vi "Generate Query.vi"(8 "error in (no error)":errorcluster, 11 "Cluster In":T1={"From Date"=timestamp(0 s since 1904-01-01), "To Date"=timestamp(0 s since 1904-01-01), "Selected Database"="", "Selected Table"="", "Selected Field"="", "Field Data"="", "DB Connection Ststus"="", "User Instruction"="", "All/ Top 1000"=FALSE, "Table Data"=[], "Query"="", "Selected Server"="", "Connection Status"=FALSE, "User ID"="", "Password"="", "Date/Field"=FALSE, "(Date/Field/All)"=enum."False", "First Run"=TRUE, "Selected DB Tables"=[], "From Date Field"="", "To Date Field"="", "Selected Table Fields"=[], "Search Type"="", "Reference"={"Top 1000/ All"=refnum, "Search by date"=refnum, "From Date"=refnum, "Select Field"=refnum, "Field Data"=refnum, "To Date"=refnum, "Tables"=refnum, "Search Type"=refnum}, "Mahine RUN Time"=0.0, "Pass/Fail querry"=""}) -> (0 "error out":errorcluster, 3 "Cluster Out":T1={"From Date"=timestamp(0 s since 1904-01-01), "To Date"=timestamp(0 s since 1904-01-01), "Selected Database"="", "Selected Table"="", "Selected Field"="", "Field Data"="", "DB Connection Ststus"="", "User Instruction"="", "All/ Top 1000"=FALSE, "Table Data"=[], "Query"="", "Selected Server"="", "Connection Status"=FALSE, "User ID"="", "Password"="", "Date/Field"=FALSE, "(Date/Field/All)"=enum."False", "First Run"=TRUE, "Selected DB Tables"=[], "From Date Field"="", "To Date Field"="", "Selected Table Fields"=[], "Search Type"="", "Reference"={"Top 1000/ All"=refnum, "Search by date"=refnum, "From Date"=refnum, "Select Field"=refnum, "Field Data"=refnum, "To Date"=refnum, "Tables"=refnum, "Search Type"=refnum}, "Mahine RUN Time"=0.0, "Pass/Fail querry"=""})   [LabVIEW 2017]
uses:
  Controls/Main Cluster.ctl
  Controls/GUI Reference Cluster.ctl
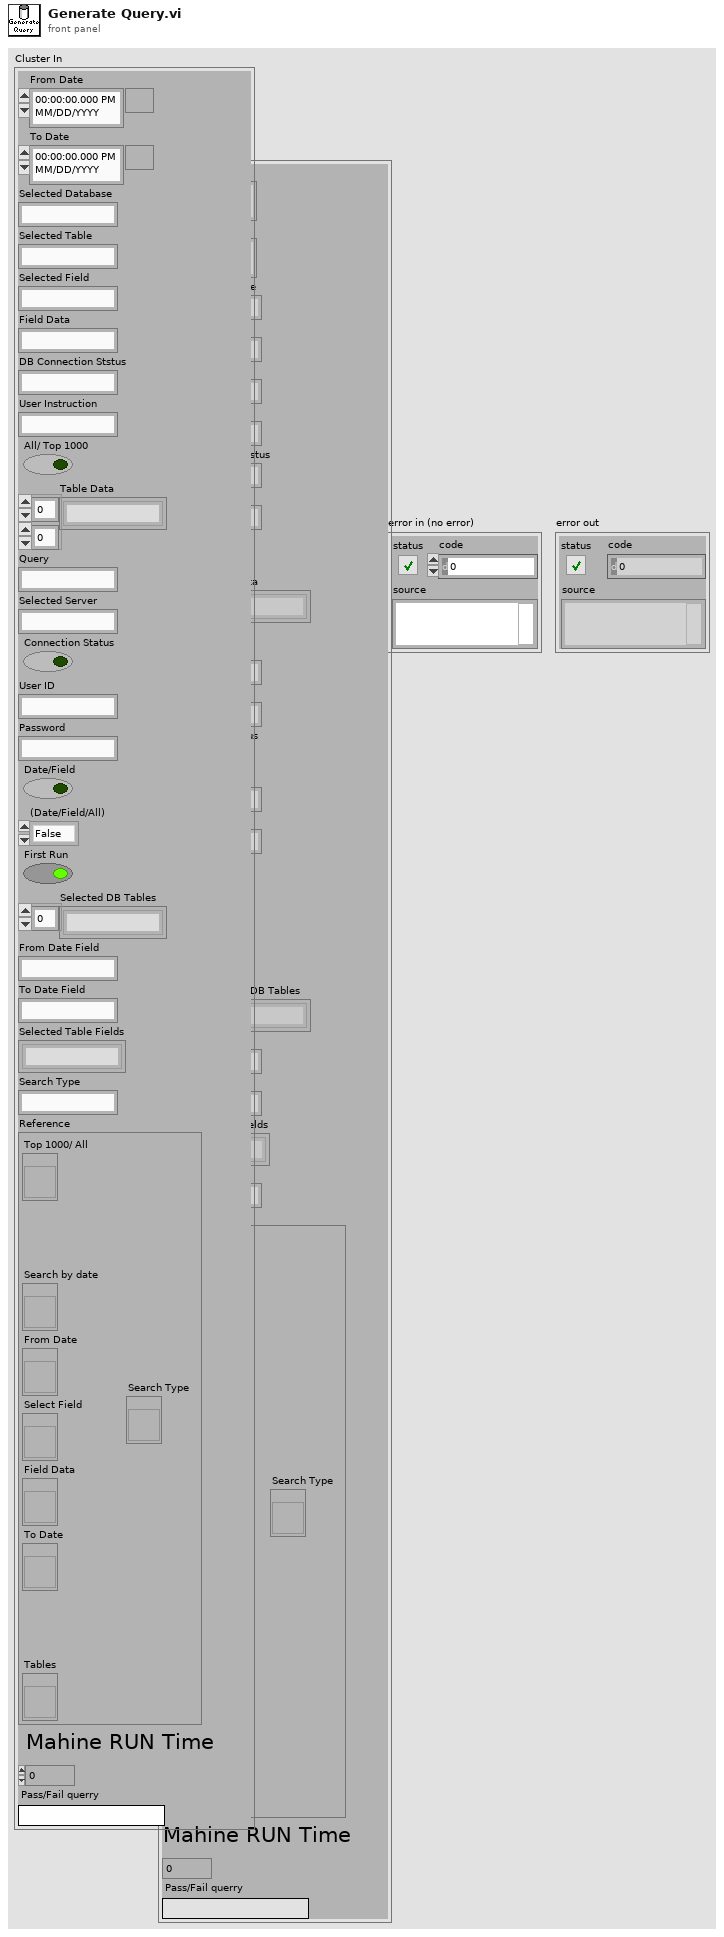
[diagram p1: front panel]
types:
  T1 = typedef "Main Cluster.ctl" = cluster{"From Date":timestamp, "To Date":timestamp, "Selected Database":string, "Selected Table":string, "Selected Field":string, "Field Data":string, "DB Connection Ststus":string, "User Instruction":string, "All/ Top 1000":bool, "Table Data":string[][], "Query":string, "Selected Server":string, "Connection Status":bool, "User ID":string, "Password":string, "Date/Field":bool, "(Date/Field/All)":enum8{"False", "True", "Mixed"}, "First Run":bool, "Selected DB Tables":string[], "From Date Field":string, "To Date Field":string, "Selected Table Fields":string[], "Search Type":string, "Reference":T2, "Mahine RUN Time":dbl, "Pass/Fail querry":string}
  T2 = typedef "GUI Reference Cluster.ctl" = cluster{"Top 1000/ All":refnum<vi>, "Search by date":refnum<vi>, "From Date":refnum<vi>, "Select Field":refnum<vi>, "Field Data":refnum<vi>, "To Date":refnum<vi>, "Tables":refnum<vi>, "Search Type":refnum<vi>}
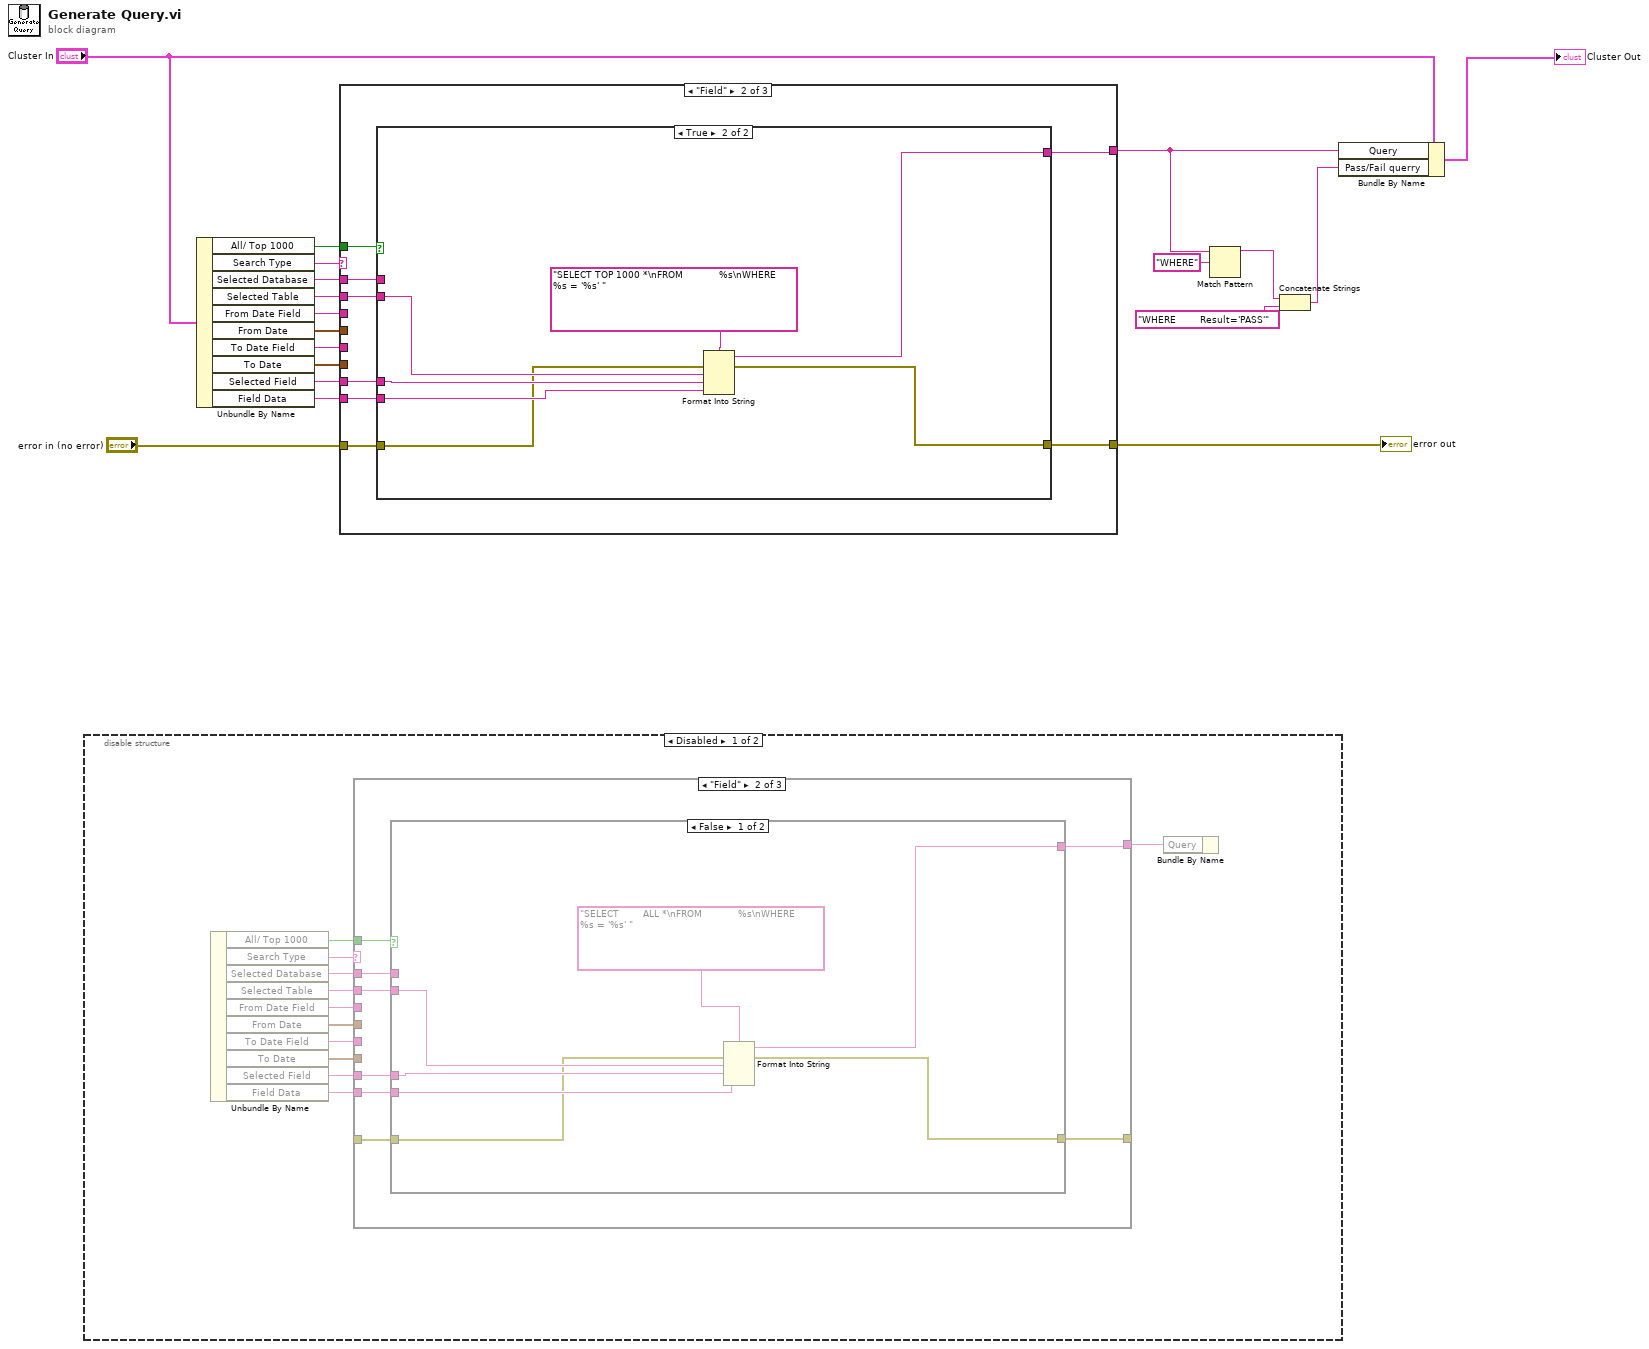
[diagram p0: block diagram]
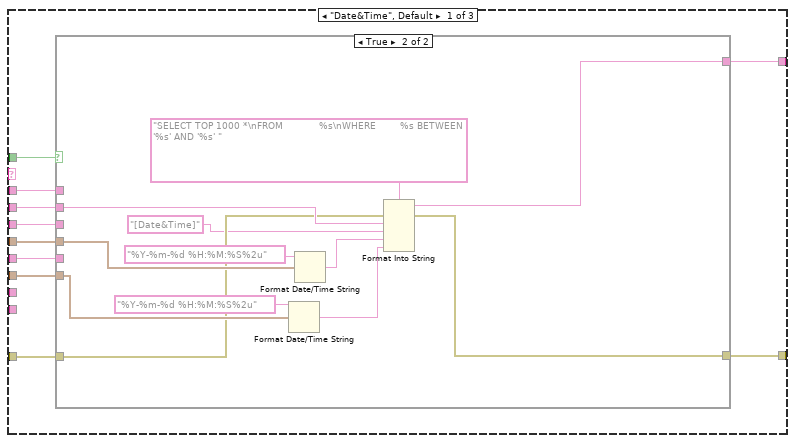
[diagram p2: hidden frame]
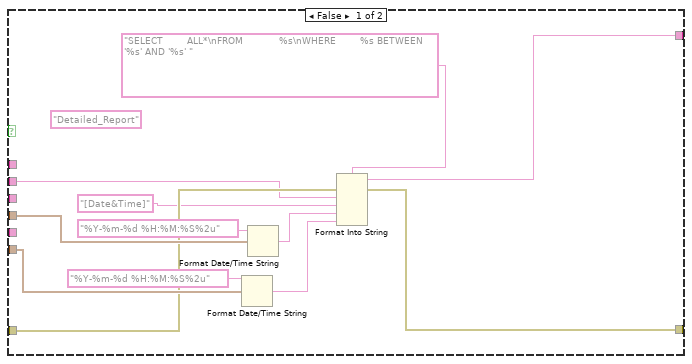
[diagram p3: hidden frame]
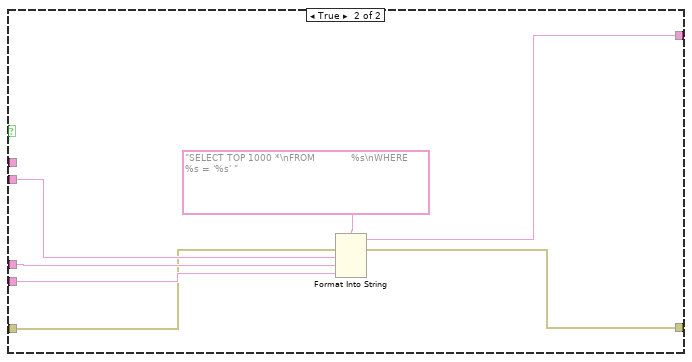
[diagram p4: hidden frame]
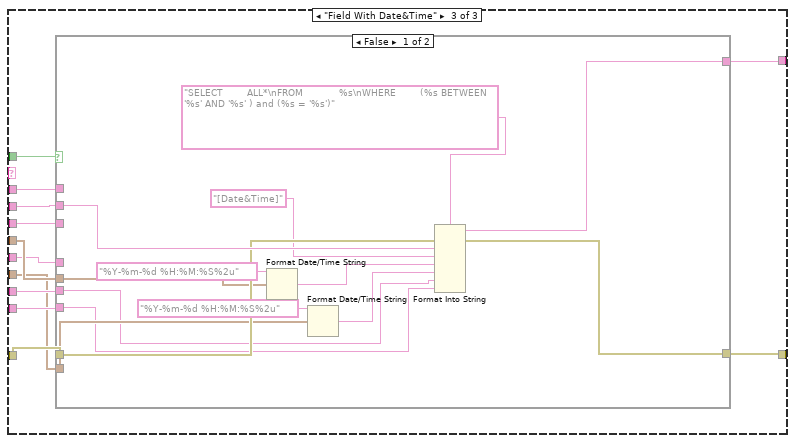
[diagram p5: hidden frame]
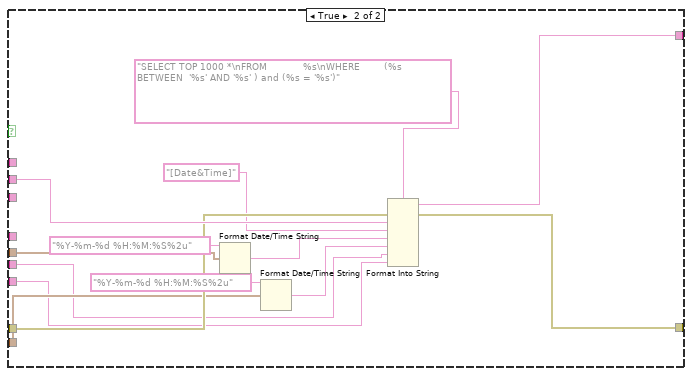
[diagram p6: hidden frame]
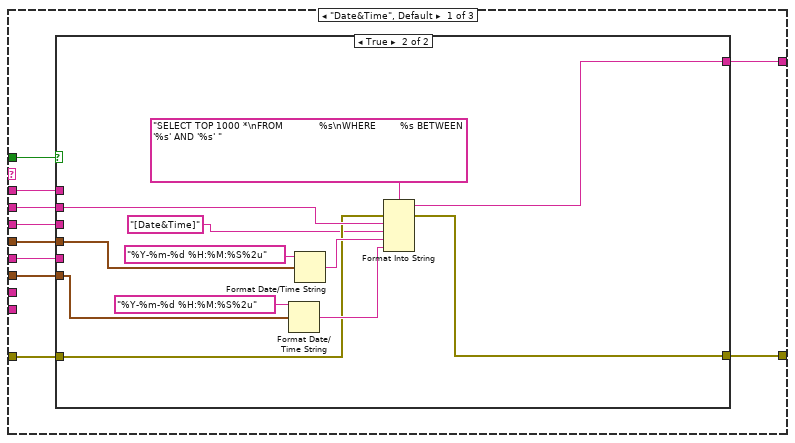
[diagram p8: hidden frame]
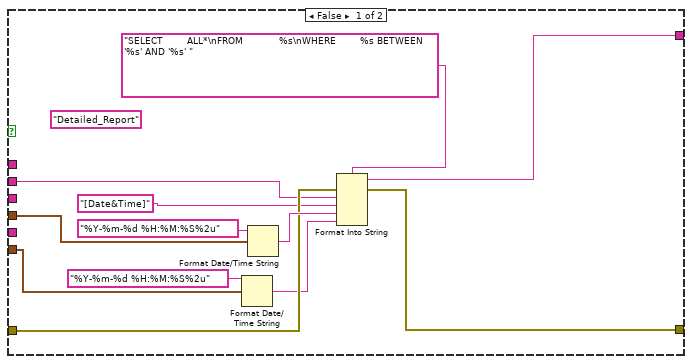
[diagram p9: hidden frame]
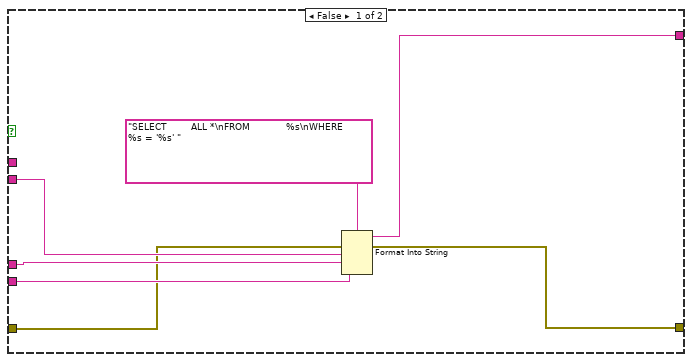
[diagram p10: hidden frame]
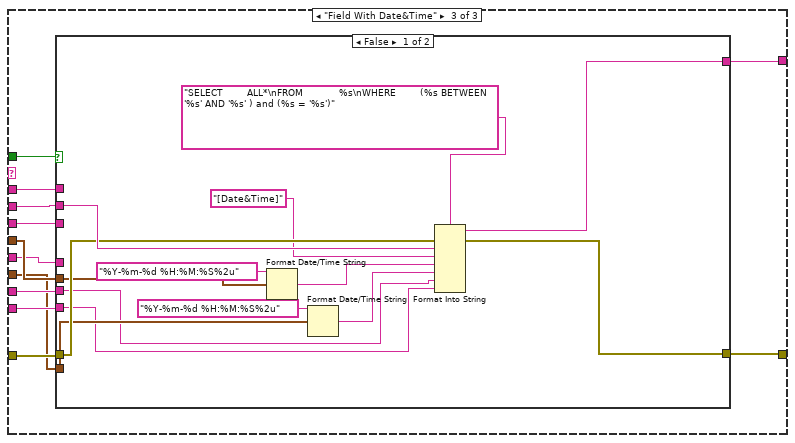
[diagram p11: hidden frame]
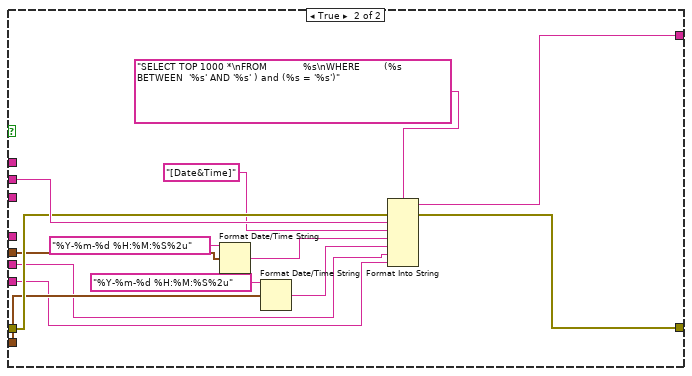
[diagram p12: hidden frame]
diagram:
  n1 = disable-structure shown="Disabled" {
    frame Disabled {
      n2 = Unbundle By Name() -> ("All/ Top 1000"=w21:bool, "Search Type"=w20:string, "Selected Database"=w23:string, "Selected Table"=w24:string, "From Date Field"=w25:string, "From Date"=w26:timestamp, "To Date Field"=w27:string, "To Date"=w28:timestamp, "Selected Field"=w30:string, "Field Data"=w31:string)  [unwired: 1 in]
      n3 = case shown="\"Field\"" w20 {
        tunnel: w21 -> [w42 w70 w98]
        tunnel: w23 -> [w41 w74 w96]
        tunnel: w24 -> [w40 w73 w95]
        tunnel: w25 -> [w39 _ w92]
        tunnel: w26 -> [w38 _ w91]
        tunnel: w27 -> [w37 _ w90]
        tunnel: w28 -> [w36 _ w89]
        tunnel: [w35 w69 w100] -> w29
        tunnel: w30 -> [_ w72 w94]
        tunnel: w31 -> [_ w71 w93]
        tunnel: [w34 w68 w97] -> w32
        tunnel: [w33 w67 w99] -> _
        frame "Date&Time", Default {
          n4 = case shown="True" w42 {
            tunnel: w41 -> [_ _]
            tunnel: w40 -> [w43 w66]
            tunnel: w39 -> [_ _]
            tunnel: w38 -> [w54 w65]
            tunnel: w37 -> [_ _]
            tunnel: w36 -> [w50 w61]
            tunnel: [w49 w59] -> w35
            tunnel: w34 -> [w48 w58]
            tunnel: [w47 w57] -> w33
            frame False {
              (unwired) "Detailed_Report"
              n5 = Format Date/Time String(time format string (%c)="%Y-%m-%d %H:%M:%S%2u", seconds (now)=w50) -> (date/time string=w44:string)  [unwired: 1 in]
              n6 = Format Date/Time String(time format string (%c)="%Y-%m-%d %H:%M:%S%2u", seconds (now)=w54) -> (date/time string=w52:string)  [unwired: 1 in]
              n7 = Format Into String(format string="SELECT        ALL*\nFROM            %s\nWHERE        %s BETWEEN  '%s' AND '%s' ", error in=w48, w43, "[Date&Time]", w52, w44) -> (resulting string=w49:string, error out=w47:errorcluster)  [unwired: 1 in]
            }
            frame True {
              n8 = Format Date/Time String(time format string (%c)="%Y-%m-%d %H:%M:%S%2u", seconds (now)=w61) -> (date/time string=w60:string)  [unwired: 1 in]
              n9 = Format Date/Time String(time format string (%c)="%Y-%m-%d %H:%M:%S%2u", seconds (now)=w65) -> (date/time string=w63:string)  [unwired: 1 in]
              n10 = Format Into String(format string="SELECT TOP 1000 *\nFROM            %s\nWHERE        %s BETWEEN  '%s' AND '%s' ", error in=w58, w66, "[Date&Time]", w63, w60) -> (resulting string=w59:string, error out=w57:errorcluster)  [unwired: 1 in]
            }
          }
        }
        frame "Field" {
          n11 = case shown="False" w70 {
            tunnel: [w81 w88] -> w69
            tunnel: w74 -> [_ _]
            tunnel: w73 -> [w80 w87]
            tunnel: w72 -> [w79 w86]
            tunnel: w71 -> [w78 w85]
            tunnel: w68 -> [w77 w84]
            tunnel: [w76 w83] -> w67
            frame False {
              n12 = Format Into String(format string="SELECT        ALL *\nFROM            %s\nWHERE        %s = '%s' ", error in=w77, w80, w79, w78) -> (resulting string=w81:string, error out=w76:errorcluster)  [unwired: 1 in]
            }
            frame True {
              n13 = Format Into String(format string="SELECT TOP 1000 *\nFROM            %s\nWHERE        %s = '%s' ", error in=w84, w87, w86, w85) -> (resulting string=w88:string, error out=w83:errorcluster)  [unwired: 1 in]
            }
          }
        }
        frame "Field With Date&Time" {
          n14 = case shown="False" w98 {
            tunnel: [w114 w128] -> w100
            tunnel: w96 -> [_ _]
            tunnel: w95 -> [w113 w127]
            tunnel: w94 -> [w102 w116]
            tunnel: w93 -> [w101 w115]
            tunnel: w97 -> [w112 w126]
            tunnel: [w111 w125] -> w99
            tunnel: w92 -> [_ _]
            tunnel: w91 -> [w110 w124]
            tunnel: w90 -> [_ _]
            tunnel: w89 -> [w106 w120]
            frame False {
              n15 = Format Date/Time String(time format string (%c)="%Y-%m-%d %H:%M:%S%2u", seconds (now)=w110) -> (date/time string=w108:string)  [unwired: 1 in]
              n16 = Format Date/Time String(time format string (%c)="%Y-%m-%d %H:%M:%S%2u", seconds (now)=w106) -> (date/time string=w105:string)  [unwired: 1 in]
              n17 = Format Into String(format string="SELECT        ALL*\nFROM            %s\nWHERE        (%s BETWEEN  '%s' AND '%s' ) and (%s = '%s')", error in=w112, w113, "[Date&Time]", w108, w105, w102, w101) -> (resulting string=w114:string, error out=w111:errorcluster)  [unwired: 1 in]
            }
            frame True {
              n18 = Format Date/Time String(time format string (%c)="%Y-%m-%d %H:%M:%S%2u", seconds (now)=w124) -> (date/time string=w122:string)  [unwired: 1 in]
              n19 = Format Date/Time String(time format string (%c)="%Y-%m-%d %H:%M:%S%2u", seconds (now)=w120) -> (date/time string=w119:string)  [unwired: 1 in]
              n20 = Format Into String(format string="SELECT TOP 1000 *\nFROM            %s\nWHERE        (%s BETWEEN  '%s' AND '%s' ) and (%s = '%s')", error in=w126, w127, "[Date&Time]", w122, w119, w116, w115) -> (resulting string=w128:string, error out=w125:errorcluster)  [unwired: 1 in]
            }
          }
        }
      }
      n21 = Bundle By Name("Query"=w29) -> (w22:cluster{})  [unwired: 1 out]
    }
    frame Enabled {
    }
  }
  n22 = Unbundle By Name("Cluster In") -> ("All/ Top 1000"=w18:bool, "Search Type"=w19:string, "Selected Database"=w16:string, "Selected Table"=w15:string, "From Date Field"=w14:string, "From Date"=w13:timestamp, "To Date Field"=w12:string, "To Date"=w11:timestamp, "Selected Field"=w10:string, "Field Data"=w9:string)
  n23 = case shown="\"Field\"" w19 {
    tunnel: w18 -> [w138 w166 w194]
    tunnel: w16 -> [w137 w170 w192]
    tunnel: w15 -> [w136 w169 w191]
    tunnel: w14 -> [w135 _ w188]
    tunnel: w13 -> [w134 _ w187]
    tunnel: w12 -> [w133 _ w186]
    tunnel: w11 -> [w132 _ w185]
    tunnel: [w131 w165 w196] -> w5
    tunnel: w10 -> [_ w168 w190]
    tunnel: w9 -> [_ w167 w189]
    tunnel: "error in (no error)" -> [w130 w164 w193]
    tunnel: [w129 w163 w195] -> w7
    frame "Date&Time", Default {
      n24 = case shown="True" w138 {
        tunnel: w137 -> [_ _]
        tunnel: w136 -> [w139 w162]
        tunnel: w135 -> [_ _]
        tunnel: w134 -> [w150 w161]
        tunnel: w133 -> [_ _]
        tunnel: w132 -> [w146 w157]
        tunnel: [w145 w155] -> w131
        tunnel: w130 -> [w144 w154]
        tunnel: [w143 w153] -> w129
        frame False {
          (unwired) "Detailed_Report"
          n25 = Format Date/Time String(time format string (%c)="%Y-%m-%d %H:%M:%S%2u", seconds (now)=w146) -> (date/time string=w140:string)  [unwired: 1 in]
          n26 = Format Date/Time String(time format string (%c)="%Y-%m-%d %H:%M:%S%2u", seconds (now)=w150) -> (date/time string=w148:string)  [unwired: 1 in]
          n27 = Format Into String(format string="SELECT        ALL*\nFROM            %s\nWHERE        %s BETWEEN  '%s' AND '%s' ", error in=w144, w139, "[Date&Time]", w148, w140) -> (resulting string=w145:string, error out=w143:errorcluster)  [unwired: 1 in]
        }
        frame True {
          n28 = Format Date/Time String(time format string (%c)="%Y-%m-%d %H:%M:%S%2u", seconds (now)=w157) -> (date/time string=w156:string)  [unwired: 1 in]
          n29 = Format Date/Time String(time format string (%c)="%Y-%m-%d %H:%M:%S%2u", seconds (now)=w161) -> (date/time string=w159:string)  [unwired: 1 in]
          n30 = Format Into String(format string="SELECT TOP 1000 *\nFROM            %s\nWHERE        %s BETWEEN  '%s' AND '%s' ", error in=w154, w162, "[Date&Time]", w159, w156) -> (resulting string=w155:string, error out=w153:errorcluster)  [unwired: 1 in]
        }
      }
    }
    frame "Field" {
      n31 = case shown="True" w166 {
        tunnel: [w177 w184] -> w165
        tunnel: w170 -> [_ _]
        tunnel: w169 -> [w176 w183]
        tunnel: w168 -> [w175 w182]
        tunnel: w167 -> [w174 w181]
        tunnel: w164 -> [w173 w180]
        tunnel: [w172 w179] -> w163
        frame False {
          n32 = Format Into String(format string="SELECT        ALL *\nFROM            %s\nWHERE        %s = '%s' ", error in=w173, w176, w175, w174) -> (resulting string=w177:string, error out=w172:errorcluster)  [unwired: 1 in]
        }
        frame True {
          n33 = Format Into String(format string="SELECT TOP 1000 *\nFROM            %s\nWHERE        %s = '%s' ", error in=w180, w183, w182, w181) -> (resulting string=w184:string, error out=w179:errorcluster)  [unwired: 1 in]
        }
      }
    }
    frame "Field With Date&Time" {
      n34 = case shown="False" w194 {
        tunnel: [w210 w224] -> w196
        tunnel: w192 -> [_ _]
        tunnel: w191 -> [w209 w223]
        tunnel: w190 -> [w198 w212]
        tunnel: w189 -> [w197 w211]
        tunnel: w193 -> [w208 w222]
        tunnel: [w207 w221] -> w195
        tunnel: w188 -> [_ _]
        tunnel: w187 -> [w206 w220]
        tunnel: w186 -> [_ _]
        tunnel: w185 -> [w202 w216]
        frame False {
          n35 = Format Date/Time String(time format string (%c)="%Y-%m-%d %H:%M:%S%2u", seconds (now)=w206) -> (date/time string=w204:string)  [unwired: 1 in]
          n36 = Format Date/Time String(time format string (%c)="%Y-%m-%d %H:%M:%S%2u", seconds (now)=w202) -> (date/time string=w201:string)  [unwired: 1 in]
          n37 = Format Into String(format string="SELECT        ALL*\nFROM            %s\nWHERE        (%s BETWEEN  '%s' AND '%s' ) and (%s = '%s')", error in=w208, w209, "[Date&Time]", w204, w201, w198, w197) -> (resulting string=w210:string, error out=w207:errorcluster)  [unwired: 1 in]
        }
        frame True {
          n38 = Format Date/Time String(time format string (%c)="%Y-%m-%d %H:%M:%S%2u", seconds (now)=w220) -> (date/time string=w218:string)  [unwired: 1 in]
          n39 = Format Date/Time String(time format string (%c)="%Y-%m-%d %H:%M:%S%2u", seconds (now)=w216) -> (date/time string=w215:string)  [unwired: 1 in]
          n40 = Format Into String(format string="SELECT TOP 1000 *\nFROM            %s\nWHERE        (%s BETWEEN  '%s' AND '%s' ) and (%s = '%s')", error in=w222, w223, "[Date&Time]", w218, w215, w212, w211) -> (resulting string=w224:string, error out=w221:errorcluster)  [unwired: 1 in]
        }
      }
    }
  }
  "error out" <- w7
  n41 = Match Pattern(string=w5, regular expression="WHERE") -> (before substring=w3:string)  [unwired: 1 in, 3 out]
  n42 = Concatenate Strings(w3, "WHERE        Result='PASS'" ("string")) -> (w1:string)
  n43 = Bundle By Name(cluster="Cluster In", "Query"=w5, "Pass/Fail querry"=w1) -> (→"Cluster Out":T1)
